vi "Moving_Avg_2.vi"(6 "Avg In":i64, 7 "It In":i64, 8 "Array In":dbl[](array[numeric]), 9 "Input":dbl) -> (0 "Avg Out":dbl format="%0.2f", 1 "It Out":i64, 2 "Array Out":dbl[](array[numeric]))   [LabVIEW 2014]
uses:
  <vilib>/Analysis/baseanly.llb/Mean (DBL).vi
  <vilib>/Analysis/NI_AALBase.lvlib
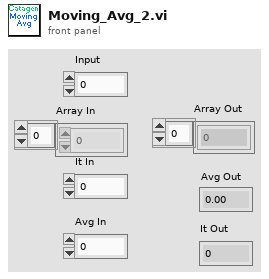
[diagram p1: front panel]
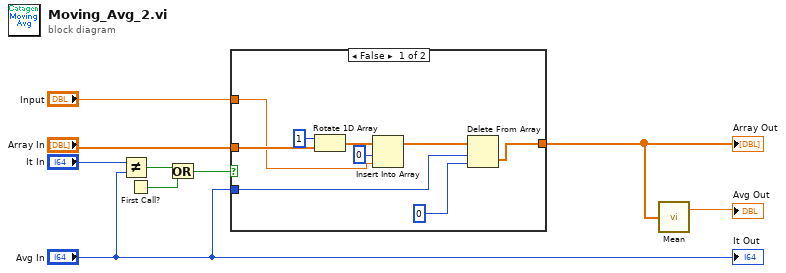
[diagram p0: block diagram]
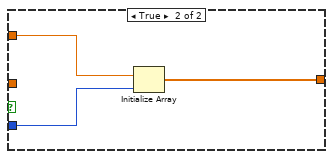
[diagram p2: hidden frame]
diagram:
  n1 = Not Equal?(x="It In", y="Avg In") -> (x != y?=w6:bool)
  n2 = First Call?() -> (First Call?: T/F=w5:bool)
  n3 = Or(x=w6, y=w5) -> (x .or. y?=w7:bool)
  n4 = case shown="False" w7 {
    tunnel: "Avg In" -> [w13 w21]
    tunnel: "Input" -> [w14 w20]
    tunnel: [w11 w19] -> w9
    tunnel: "Array In" -> [w18 _]
    frame False {
      n5 = Rotate 1D Array(1:w18, 2:1 ("n")) -> (0:w17:dbl[])
      n6 = Insert Into Array(array=w17, index=0, new element=w14) -> (w10:dbl[])
      n7 = Delete From Array(array=w10, length=w13, index=0) -> (deleted portion=w11:dbl[])  [unwired: 1 out]
    }
    frame True {
      n8 = Initialize Array "Initialize Array"(w20, w21) -> (w19:dbl[])
    }
  }
  "Array Out" <- w9
  n9 = call-poly <vilib>:"Mean.vi"("X"=w9) -> ("mean"=→"Avg Out":dbl)  [unwired: 1 out]
  "It Out" <- "Avg In"
